vi "i2c_read_status.vi"(0 "I2C interface":T4, 1 "Start index":i32, 4 "Filter":T1, 5 "error in":errorcluster) -> (16 "End index":i32, 18 "Result":T3[](array[typedef]), 19 "error out":errorcluster)   [LabVIEW 2014]
uses:
  i2c_interface.ctl
  fpga_reference.ctl
  i2c_status_cluster.ctl
  Common/i2c_status.ctl
  status_filter.ctl
  <vilib>/Utility/error.llb/Error Cluster From Error Code.vi
  <vilib>/rvi/errors/niLvFpgaAdjustHostInterfaceError.vi
  <vilib>/rvi/interface/nirviMethod/nirviMethod.xnode
  FPGA Bitfiles/i2cmuxdemux.lvbitx
  <vilib>/FPGAPlugInAG/PCIe-7842R/niLvFpga_ReadFifo_PCIe-7842R.vi
  <vilib>/rvi/errors/niLvFpgaMergeErrorWithErrorCode.vi
panel:
  in  "Buffer length":i32=20000
  out "Elements Remaining":u32
  # "The index to start returning filtered status at, normally the preceding end index."
  # "Total number of status events recieved.\nThis is cumulative (does not wrap.)"
  # "When filtering the code, the comparison\nmay be = or >=, according to the flag."
  # "For argument and bus, if the filter value is \nnegative, then the filter is disabled, otherwise\nthe value is compared with =."
  # "Read status from I2C controller.  Any current status goes into a ring buffer, and then we also generate a result of filtered status events.   This must be called periodically to poll for new status, and is also used to access status events from the buffer."
  # "Locals:"
  # "Length of ring-buffer (in records.)"
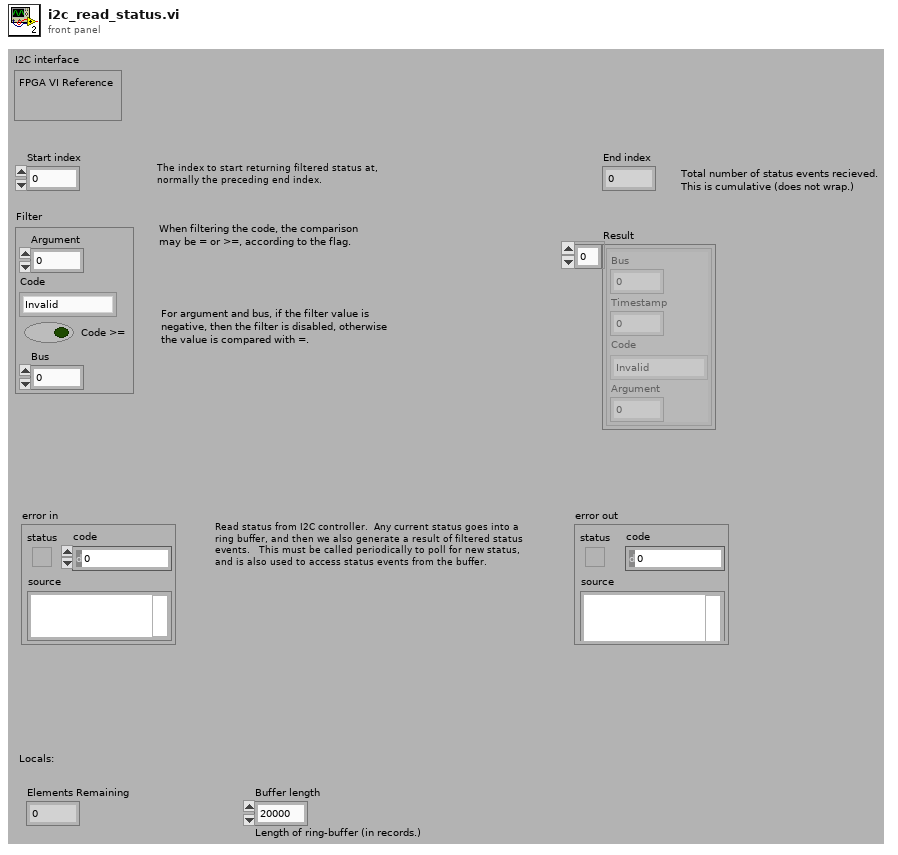
[diagram p1: front panel]
types:
  T1 = typedef "status_filter.ctl" = cluster{"Argument":i16, "Code":T2, "Code >=":bool, "Bus":i16}
  T2 = typedef "i2c_status.ctl" = enum8{"Invalid", "Command", "I2C start", "Trigger wait", "TX data wait", "Sequence", "Receive data", "I2C error", "Address NACK", "Data NACK", "SDA stuck", "SCL stuck", "Bad command"}
  T3 = typedef "i2c_status_cluster.ctl" = cluster{"Bus":u8, "Timestamp":u16, "Code":T2, "Argument":u8}
  T4 = typedef "i2c_interface.ctl" = cluster{"FPGA VI Reference":T5}
  T5 = typedef "fpga_reference.ctl" = refnum<k20>
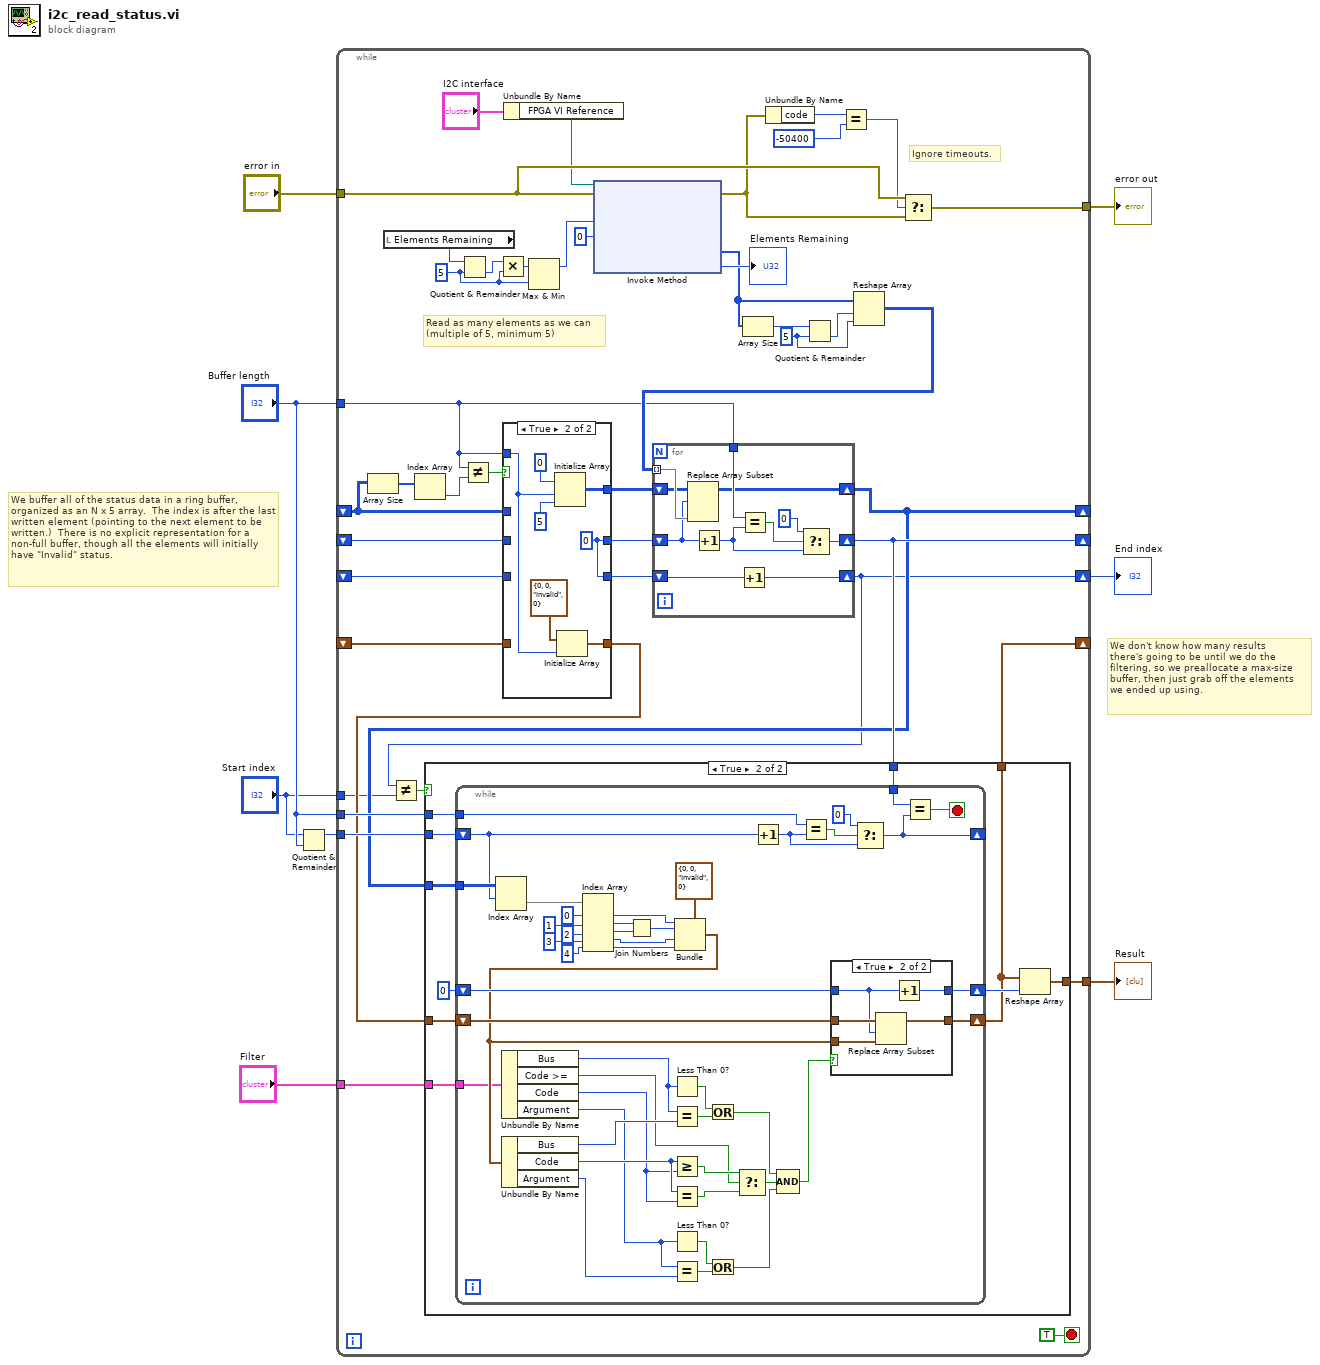
[diagram p0: block diagram]
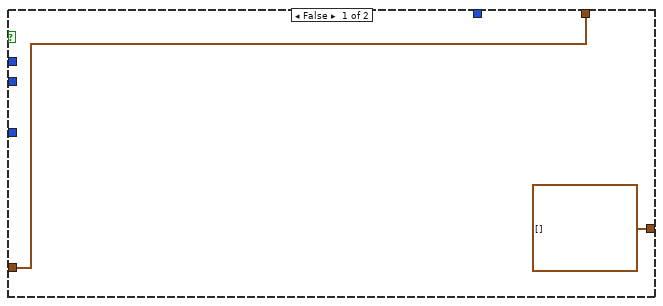
[diagram p2: hidden frame]
diagram:
  # "We don't know how many results\nthere's going to be until we do the \nfiltering, so we preallocate a max-size\nbuffer, then just grab off the elements\nwe ended up using."
  # "We buffer all of the status data in a ring buffer, organized as an N x 5 array.  The index is after the last written element (pointing to the next element to be written.)  There is no explicit representation for a non-full buffer, though all the elements will initially have \"Invalid\" status."
  n1 = Quotient & Remainder(x="Start index", y="Buffer length") -> (x-y*floor(x/y)=w5:i32)  [unwired: 1 out]
  n2 = while {
    shift-right: [w17] -> _
    shift-left: _ -> [w29]
    shift-right: [w18] -> _
    shift-left: _ -> [w28]
    tunnel: "error in" -> [w51]
    tunnel: [w50] -> w7
    tunnel: "Buffer length" -> [w23]
    shift-right: [w12] -> w6
    shift-left: _ -> [w22]
    tunnel: w5 -> [w20]
    tunnel: "Buffer length" -> [w19]
    shift-right: [w15] -> _
    shift-left: _ -> [w16]
    tunnel: [w10] -> w3
    tunnel: "Start index" -> [w13]
    tunnel: "Filter" -> [w9]
    stop <- TRUE stop-if-true
    w30 = 5 ("y")
    w38 = u32 5 ("y")
    # "Read as many elements as we can\n(multiple of 5, minimum 5)"
    # "Ignore timeouts."
    n3 = Array Size(array=w29) -> (size(s)=w35:i32[])
    n4 = local read "Elements Remaining"() -> (w40:u32)
    n5 = Index Array(array=w35) -> (element=w34:i32)  [unwired: 1 in]
    n6 = Quotient & Remainder(x=w40, y=w38) -> (floor(x/y)=w36:u32)  [unwired: 1 out]
    n7 = Not Equal?(x=w23, y=w34) -> (x != y?=w33:bool)
    n8 = Multiply(x=w36, y=w38) -> (x*y=w39:u32)
    n9 = case shown="True" w33 {
      tunnel: w23 -> [_ w132]
      tunnel: [w129 w136] -> w27
      tunnel: w29 -> [w129 _]
      tunnel: w28 -> [w130 _]
      tunnel: [w130 w134] -> w25
      tunnel: w22 -> [w128 _]
      tunnel: [w128 w134] -> w21
      tunnel: [w127 w131] -> w14
      tunnel: w16 -> [w127 _]
      frame False {
      }
      frame True {
        w134 = 0 ("Buffer length")
        n10 = Initialize Array(u8 0, w132, 5 ("dimension size")) -> (w136:u8[][])
        n11 = Initialize Array(T3 {"Bus"=0, "Timestamp"=0, "Code"=enum."Invalid", "Argument"=0} ("I2C status 2"), w132) -> (w131:T3[])
      }
    }
    n12 = Unbundle By Name("I2C interface") -> ("FPGA VI Reference"=w47:T5)
    n13 = Max & Min(x=w39, y=w38) -> (max(x,y)=w37:u32)  [unwired: 1 out]
    n14 = xnode "Invoke Method"("FPGA VI Reference In"=w47, "error in"=w51, "Number of Elements"=w37, "Timeout (ms)"=0) -> ("error out"=w44:errorcluster, "Data"=w32:u8[], "Elements Remaining"=→"Elements Remaining":u32)  [unwired: 1 out]
    n15 = Array Size(array=w32) -> (size(s)=w31:i32)
    n16 = Unbundle By Name(w44) -> ("code"=w45:i32)
    n17 = Quotient & Remainder(x=w31, y=w30) -> (floor(x/y)=w26:i32)  [unwired: 1 out]
    n18 = Equal?(x=w45, y=-50400 ("code")) -> (x = y?=w42:bool)
    n19 = Reshape Array(w32, w26, w30) -> (w24:u8[][])
    n20 = for {
      tunnel: w24 -> [w126] mode=indexing
      shift-right: [w122] -> w18
      shift-left: w25 -> [w124]
      tunnel: w23 -> [w123]
      shift-right: [w118] -> w17
      shift-left: w27 -> [w125]
      shift-right: [w116] -> w12
      shift-left: w21 -> [w117]
      n21 = Replace Array Subset(array=w125, new element=w126, index (row)=w124) -> (w118:u8[][])  [unwired: 1 in]
      n22 = Increment(x=w124) -> (x+1=w119:i32)
      n23 = Increment(x=w117) -> (x+1=w116:i32)
      n24 = Equal?(x=w123, y=w119) -> (x = y?=w121:bool)
      n25 = Select(t=0 ("Buffer length"), s=w121, f=w119) -> (s? t:f=w122:i32)
    }
    n26 = Not Equal?(x=w12, y=w13) -> (x != y?=w11:bool)
    n27 = case shown="True" w11 {
      tunnel: w20 -> [_ w63]
      tunnel: w19 -> [_ w62]
      tunnel: w18 -> [_ w61]
      tunnel: w17 -> [_ w60]
      tunnel: [w52 w55] -> w15
      tunnel: w14 -> [w52 w58]
      tunnel: [T3[] [] w57] -> w10
      tunnel: w9 -> [_ w54]
      frame False {
      }
      frame True {
        n28 = while {
          shift-right: [w96] -> _
          shift-left: w63 -> [w88]
          tunnel: w62 -> [w98]
          tunnel: w61 -> [w95]
          tunnel: w60 -> [w89]
          shift-right: [w82] -> w56
          shift-left: 0 ("Buffer length") -> [w85]
          shift-right: [w84] -> w55
          shift-left: w58 -> [w86]
          tunnel: w54 -> [w68]
          stop <- w108 stop-if-true
          n29 = Index Array(array=w89, index (row)=w88) -> (element=w87:u8[])  [unwired: 1 in]
          n30 = Unbundle By Name(w68) -> ("Bus"=w67:i16, "Code >="=w66:bool, "Code"=w65:T2, "Argument"=w64:i16)
          n31 = Index Array(array=w87, index #1=0 ("index"), index #2=1 ("index"), index #3=2 ("index"), index #4=3 ("index"), index #5=4 ("index")) -> (element #1=w94:u8, element #2=w102:u8, element #3=w101:u8, element #4=w92:u8, element #5=w91:u8)
          n32 = Join Numbers(hi=w102, lo=w101) -> ((hi.lo)=w93:u16)
          n33 = Less Than 0?(x=w67) -> (x < 0?=w80:bool)
          n34 = Less Than 0?(x=w64) -> (x < 0?=w77:bool)
          n35 = Bundle(cluster=T3 {"Bus"=0, "Timestamp"=0, "Code"=enum."Invalid", "Argument"=0} ("I2C status 2"), "Bus"=w94, "Timestamp"=w93, "Code"=w92, "Argument"=w91) -> (w83:T3)
          n36 = Unbundle By Name(w83) -> ("Bus"=w81:u8, "Code"=w69:T2, "Argument"=w76:u8)
          n37 = Equal?(x=w67, y=w81) -> (x = y?=w79:bool)
          n38 = Greater Or Equal?(x=w69, y=w65) -> (x >= y?=w75:bool)
          n39 = Equal?(x=w69, y=w65) -> (x = y?=w74:bool)
          n40 = Equal?(x=w64, y=w76) -> (x = y?=w78:bool)
          n41 = Or(x=w80, y=w79) -> (x .or. y?=w73:bool)
          n42 = Or(x=w77, y=w78) -> (x .or. y?=w71:bool)
          n43 = Select(t=w75, s=w66, f=w74) -> (s? t:f=w72:bool)
          n44 = Increment(x=w88) -> (x+1=w97:i32)
          n45 = Compound Arithmetic op=AND(w73, w72, w71) -> (w70:bool)
          n46 = Equal?(x=w98, y=w97) -> (x = y?=w99:bool)
          n47 = case shown="True" w70 {
            tunnel: w86 -> [w110 w115]
            tunnel: w85 -> [w109 w112]
            tunnel: [w110 w114] -> w84
            tunnel: w83 -> [_ w113]
            tunnel: [w109 w111] -> w82
            frame False {
            }
            frame True {
              n48 = Replace Array Subset(array=w115, new element=w113, index=w112) -> (w114:T3[])
              n49 = Increment(x=w112) -> (x+1=w111:i32)
            }
          }
          n50 = Select(t=0 ("Buffer length"), s=w99, f=w97) -> (s? t:f=w96:i32)
          n51 = Equal?(x=w95, y=w96) -> (x = y?=w108:bool)
        }
        n52 = Reshape Array(w55, w56) -> (w57:T3[])
      }
    }
    n53 = Select(t=w51, s=w42, f=w44) -> (s? t:f=w50:errorcluster)
  }
  "error out" <- w7
  "End index" <- w6
  "Result" <- w3
